vi "intersect_edge.vi"(9 "Dim Num":i32, 10 "check value":sgl, 11 "edge":cluster{"array":sgl[], "array 2":sgl[]}) -> (2 "In Range?":bool, 3 "Output Point":T1)   [LabVIEW 2020, in "3DPC_SurfacePlot.xctl"]
uses:
  <vilib>/Native 3D Graph/xcontrol/3DPC_SurfacePlot.xctl
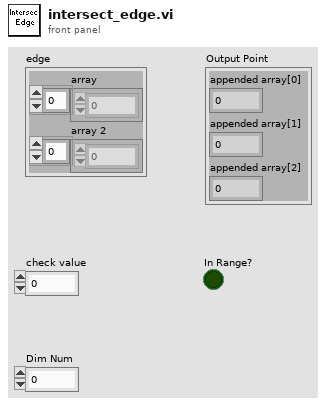
[diagram p1: front panel]
types:
  T1 = cluster{"appended array[0]":sgl, "appended array[1]":sgl, "appended array[2]":sgl}
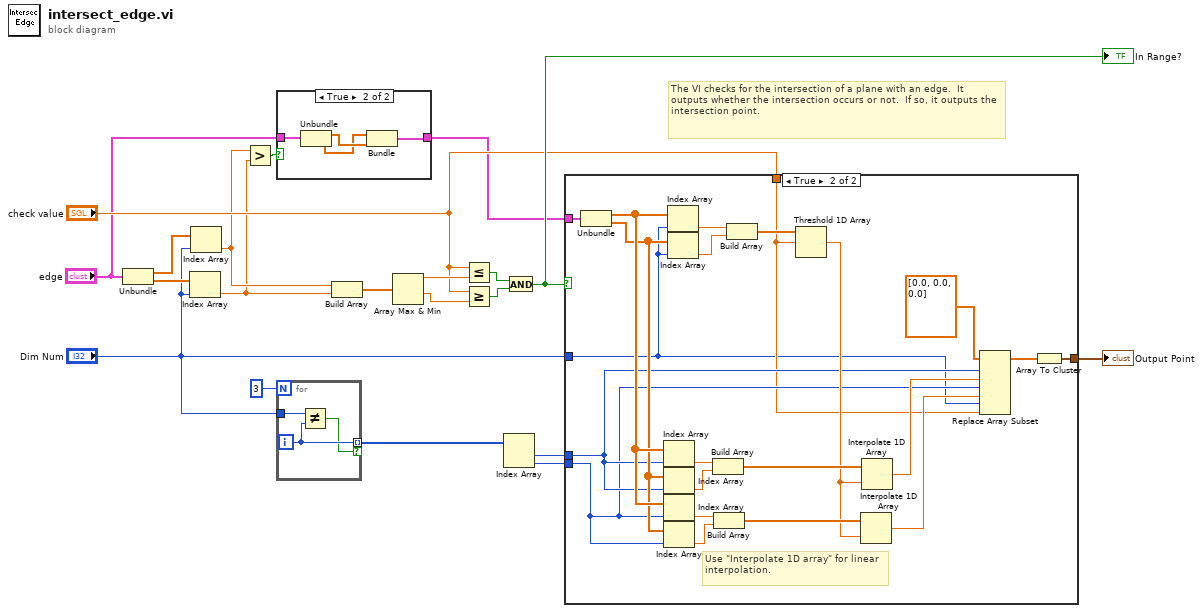
[diagram p0: block diagram]
diagram:
  # "The VI checks for the intersection of a plane with an edge.  It outputs whether the intersection occurs or not.  If so, it outputs the intersection point."
  n1 = Unbundle("edge") -> ("array"=w20:sgl[], "array 2"=w19:sgl[])
  n2 = Index Array(array=w19, index="Dim Num") -> (element=w5:sgl)
  n3 = Index Array(array=w20, index="Dim Num") -> (element=w6:sgl)
  n4 = Greater?(x=w6, y=w5) -> (0:w4:bool)
  n5 = case shown="True" w4 {
    tunnel: "edge" -> [w21 w25]
    tunnel: [w21 w22] -> w2
    frame False {
    }
    frame True {
      n6 = Unbundle(w25) -> ("array"=w24:sgl[], "array 2"=w23:sgl[])
      n7 = Bundle("array 2"=w23, "array"=w24) -> (w22:cluster{"array 2":sgl[], "array":sgl[]})  [unwired: 1 out]
    }
  }
  n8 = for {
    N: 3 -> [_]
    tunnel: "Dim Num" -> [w28]
    tunnel: [w27] -> w1 mode=indexing if=w26
    i -> [w27]
    n9 = Not Equal?(x=w28, y=w27) -> (x != y?=w26:bool)
  }
  n10 = Build Array(w6, w5) -> (w18:sgl[])
  n11 = Array Max & Min(array=w18) -> (max value=w16:sgl, min value=w17:sgl)  [unwired: 2 out]
  n12 = Less Or Equal?(x="check value", y=w16) -> (x <= y?=w15:bool)
  n13 = Greater Or Equal?(x="check value", y=w17) -> (x >= y?=w14:bool)
  n14 = Index Array(array=w1) -> (element #1=w11:i32, element #2=w10:i32)  [unwired: 2 in]
  n15 = And(x=w15, y=w14) -> (x .and. y?=w13:bool)
  "In Range?" <- w13
  n16 = case shown="True" w13 {
    tunnel: w2 -> [_ w50]
    tunnel: w11 -> [_ w35]
    tunnel: w10 -> [_ w33]
    tunnel: "check value" -> [_ w32]
    tunnel: "Dim Num" -> [_ w29]
    tunnel: [_ w30] -> w7
    frame False {
    }
    frame True {
      # "Use \"Interpolate 1D array\" for linear interpolation."
      n17 = Unbundle(w50) -> ("array 2"=w49:sgl[], "array"=w48:sgl[])
      n18 = Index Array(array=w49, index=w35) -> (element=w47:sgl)
      n19 = Index Array(array=w48, index=w35) -> (element=w46:sgl)
      n20 = Index Array(array=w49, index=w33) -> (element=w45:sgl)
      n21 = Index Array(array=w48, index=w33) -> (element=w44:sgl)
      n22 = Index Array(array=w49, index=w29) -> (element=w43:sgl)
      n23 = Index Array(array=w48, index=w29) -> (element=w42:sgl)
      n24 = Build Array(w47, w46) -> (w41:sgl[])
      n25 = Build Array(w45, w44) -> (w39:sgl[])
      n26 = Build Array(w43, w42) -> (w40:sgl[])
      n27 = Threshold 1D Array(2:w32, 3:w40) -> (0:w38:sgl)  [unwired: 1 out]
      n28 = Interpolate 1D Array(1:w38, 2:w39) -> (0:w34:sgl)
      n29 = Interpolate 1D Array(1:w38, 2:w41) -> (0:w36:sgl)
      n30 = Replace Array Subset(array=sgl[] [0.0, 0.0, 0.0] ("appended array"), new element #1=w36, index #1=w35, new element #2=w34, index #2=w33, new element #3=w32, index #3=w29) -> (w31:sgl[])
      n31 = Array To Cluster(array=w31) -> (cluster=w30:T1)
    }
  }
  "Output Point" <- w7
